vi "Update Bind Method Controls.vi"(8 "error in (no error)":errorcluster, 10 "Method Name":string, 11 "VI in":refnum<vi>) -> (0 "error out":errorcluster, 3 "VI out":refnum<vi>)   [LabVIEW 2019, in "gRPC Template Creation Utility.lvlib"]
uses:
  gRPC Template Creation Utility.lvlib
  <vilib>/Utility/traverseref.llb/TRef TravTarget.ctl
  <vilib>/Utility/traverseref.llb/VI Scripting - Traverse.lvlib
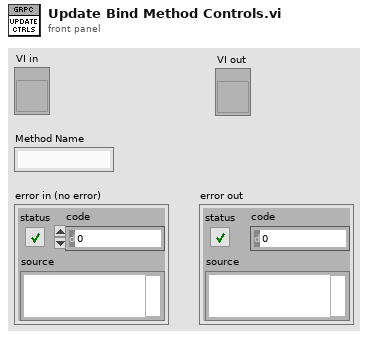
[diagram p1: front panel]
types:
  T1 = typedef "TRef TravTarget.ctl" = enum16{"FP", "BD", "Other"}
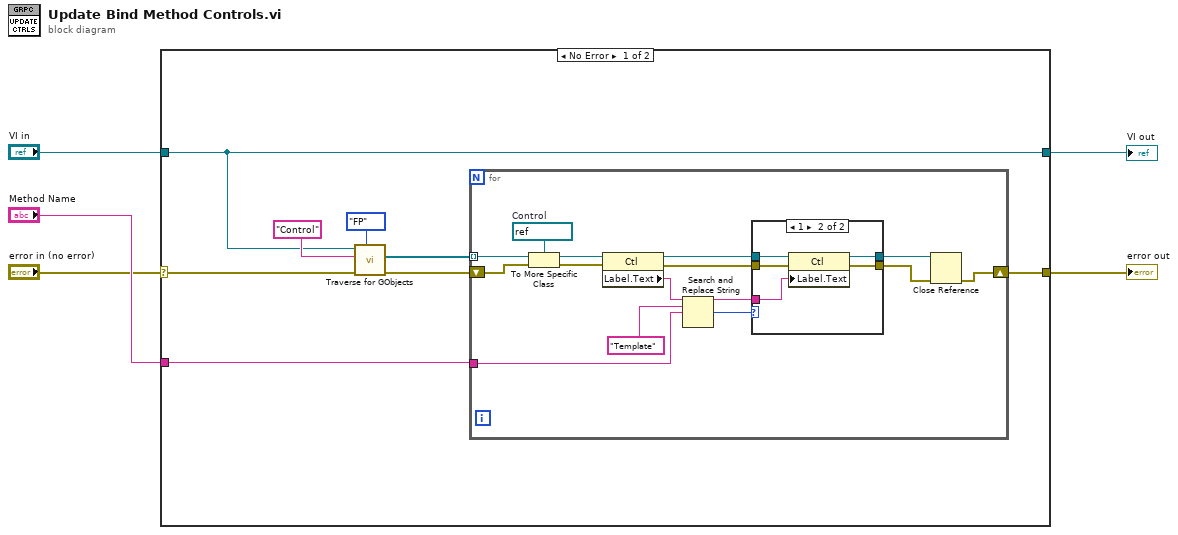
[diagram p0: block diagram]
diagram:
  n1 = case shown="No Error" "error in (no error)" {
    selector: "error in (no error)" -> [w8 w37]
    tunnel: [w13 w37] -> w5
    tunnel: "Method Name" -> [w6 _]
    tunnel: "VI in" -> [w7 w36]
    tunnel: [w7 w36] -> w1
    frame No Error {
      n2 = call <vilib>:"Traverse for GObjects.vi"("Traverse Target"=TRef_TravTarget."FP", "error in (no error)"=w8, "Class Name"="Control", "VI Refnum"=w7) -> ("error out"=w9:errorcluster, "References"=w10:refnum<vi>[])  [unwired: 4 in, 2 out]
      n3 = for {
        tunnel: w10 -> [w27] mode=indexing
        shift-right: [w17] -> w13
        shift-left: w9 -> [w26]
        tunnel: w6 -> [w22]
        w28 = refnum<vi> refnum  # Control
        n4 = To More Specific Class(target class=w28, reference=w27, error in=w26) -> (specific class reference=w25:refnum<vi>, error out=w24:errorcluster)
        n5 = property class="Ctl"(reference=w25, error in=w24) -> (reference out=w21:refnum<vi>, error out=w18:errorcluster, "Label.Text"=w14:string)
        n6 = Search and Replace String(input string=w14, search string="Template", replace string=w22) -> (result string=w15:string, number of replacements=w16:i32)  [unwired: 5 in, 2 out]
        n7 = case shown="1" w16 {
          tunnel: w21 -> [w30 w35]
          tunnel: [w30 w34] -> w20
          tunnel: [w29 w33] -> w19
          tunnel: w18 -> [w29 w32]
          tunnel: w15 -> [_ w31]
          frame 0, Default {
          }
          frame 1 {
            n8 = property class="Ctl"(reference=w35, error in=w32, "Label.Text"=w31) -> (reference out=w34:refnum<vi>, error out=w33:errorcluster)
          }
        }
        n9 = Close Reference(reference=w20, error in (no error)=w19) -> (error out=w17:errorcluster)
      }
    }
    frame Error {
    }
  }
  "error out" <- w5
  "VI out" <- w1
